vi "U8 to string.vi"() -> ()   [LabVIEW 2013]
panel:
  out "data string":string
  in  "u8 Data[]":u8[](array[numeric]) format="%.0x"
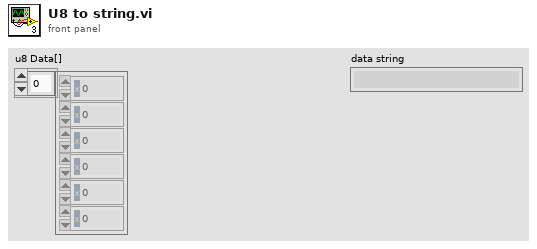
[diagram p1: front panel]
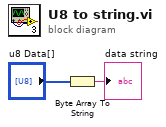
[diagram p0: block diagram]
diagram:
  n1 = Byte Array To String(unsigned byte array="u8 Data[]") -> (string=→"data string":string)
